vi "12-2.vi"() -> ()   [LabVIEW 2022 SP3, in "AoC22.lvlib"]
uses:
  AoC22.lvlib
  Map.ctl
panel:
  out "End gScore":i32
  out "Finished":bool
  out "No Solution":bool
  out "Elev":u8[][](graph)
  out "Cur":cluster{"Row":i32, "Col":i32}
  out "Numeric":i32
  out "Viz":i32[][](graph)
  in  "Speed":u32(slide)
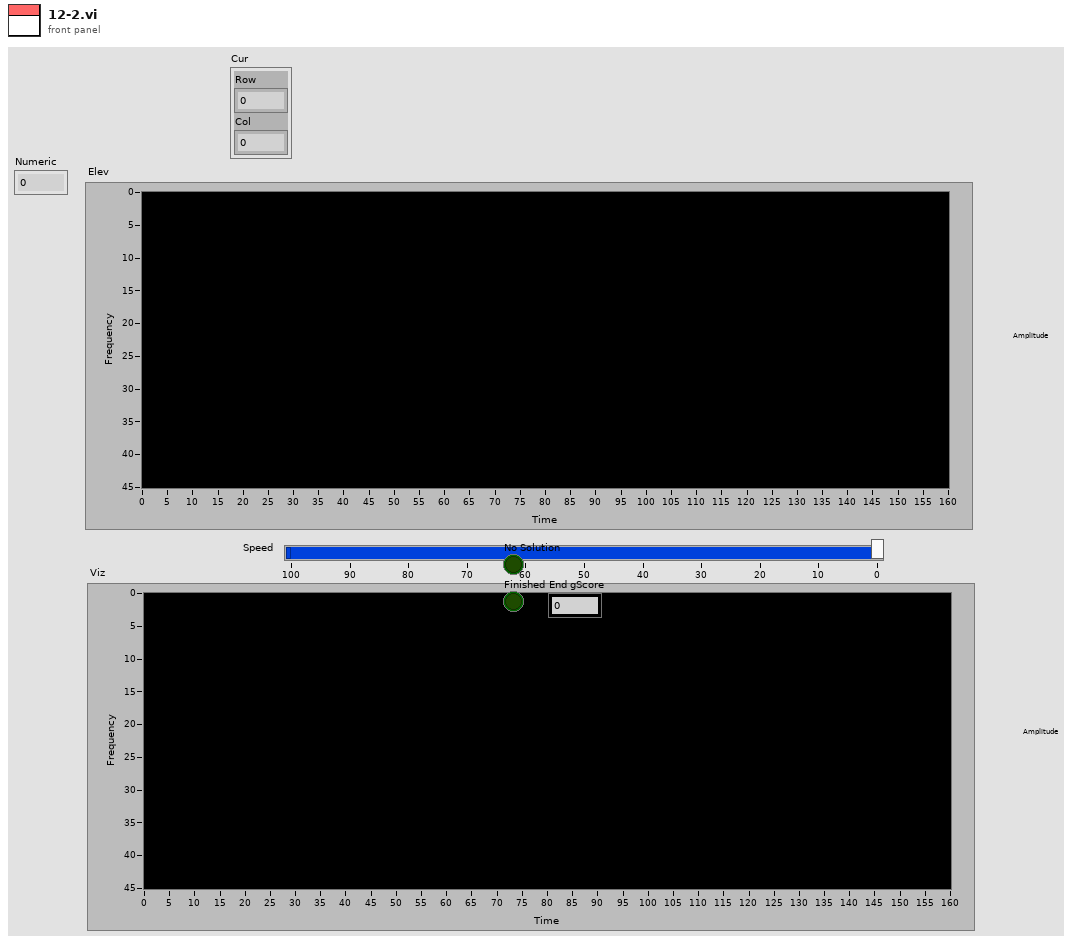
[diagram p1: front panel]
types:
  T1 = typedef "AoC22.lvlib/Map.ctl" = cluster{"Elevation":u8[][], "From":cluster{"Row":i32, "Col":i32}[][], "fScore":i32[][], "gScore":i32[][], "Start":cluster{"Row":i32, "Col":i32}, "End":cluster{"Row":i32, "Col":i32}, "openMap":map{i32, cluster{"Row":i32, "Col":i32}[]}, "openSet":set{cluster{"Row":i32, "Col":i32}}, "Vis":u8[][], "In Open":bool[][]}
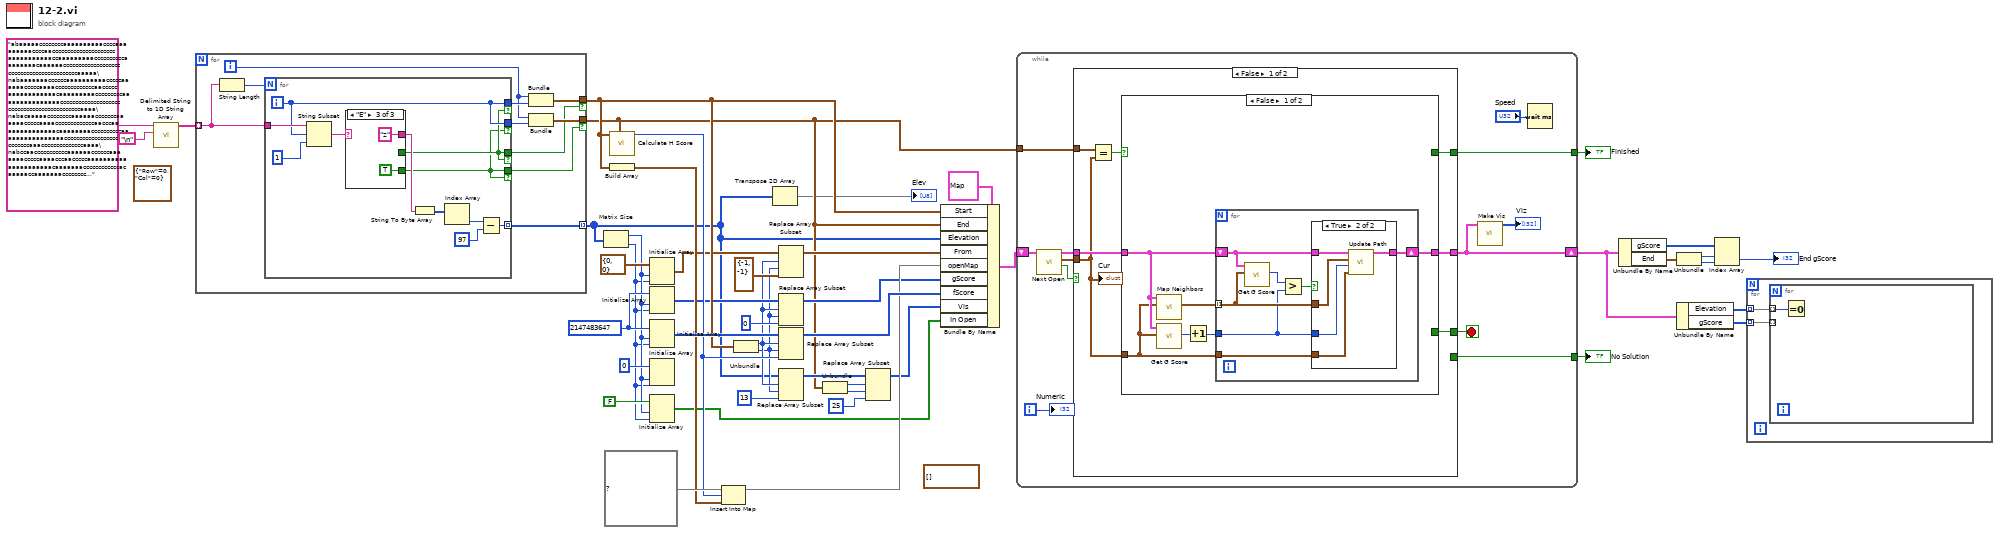
[diagram p0: block diagram]
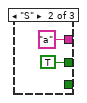
[diagram p3: hidden frame]
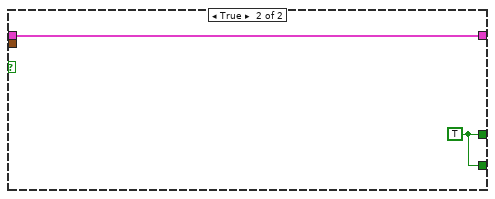
[diagram p6: hidden frame]
diagram:
  (unwired) cluster{"Row":i32, "Col":i32}[] [] ("Start")
  w37 = 2147483647 ("element")
  (unwired) cluster{"Row":i32, "Col":i32} {"Row"=0, "Col"=0}
  n1 = call <vilib>:"Delimited String to 1D String Array.vi"("delimiter"="\n", "delimited string"="abaaaaaccccccccaaaaaaaaaaccccaaaaaaaaaccccaacccccccccccccccccccccaaaaaaaaaaaccaaaaaaaaaccccccccccaaaaaaaacaaaaaaccccccccccccccccccccccccccccccccccccccccccaaaaa\nabaaaaaaaccccccaaaaaaaaaacccccaaaaaacccccaaaacccccccccccccaacccccaaaaaaaaaaaacaaaaaaaaacccccccccaaaaaaaaaaaaaaaccccccccccccccccccccccccccccccccccccccccccccaaaa\nabacaaaaaccccccccaaaaaacccccccaaaaaacccccaaaacccccccccccccaacccaaaaaaaaaaaaaacaaaaaaaaccccccccccaaaaaaaaaaaaaaaaccccccccccccccccccccccccccaaaccccccccccccccaaaa\nabccaacccccccccccaaaaaaccccccaaaaaaacccccaaaacccaacccccaaaaaaaaaaaaaaaaaaaaacaaaaaaaccccccccccccacaaaaaccaaaaaaacccccccc...") -> ("string array"=w44:string[])  [unwired: 9 in]
  n2 = for {
    tunnel: w44 -> [w55] mode=indexing
    tunnel: [w54] -> w8 mode=indexing
    tunnel: [w50] -> w34 if=w48
    tunnel: [w49] -> w13 if=w47
    i -> [w51]
    n3 = String Length(string=w55) -> (length=w56:i32)
    n4 = for {
      N: w56 -> [_]
      tunnel: w55 -> [w67]
      tunnel: [w63] -> w53 if=w62
      tunnel: [w62] -> w48 if=w62
      tunnel: [w61] -> w47 if=w61
      tunnel: [w63] -> w52 if=w61
      tunnel: [w57] -> w54 mode=indexing
      i -> [w63]
      n5 = String Subset(string=w67, offset (0)=w63, length (rest)=1 ("length (rest)")) -> (substring=w65:string)
      n6 = case shown="\"E\"" w65 {
        selector: w65 -> [w68 _ _]
        tunnel: [w68 "a" "z"] -> w64
        tunnel: [_ TRUE _] -> w62
        tunnel: [_ _ TRUE] -> w61
        frame Default {
        }
        frame "S" {
        }
        frame "E" {
        }
      }
      n7 = String To Byte Array(string=w64) -> (unsigned byte array=w60:u8[])
      n8 = Index Array(array=w60) -> (element=w59:u8)  [unwired: 1 in]
      n9 = Subtract(x=w59, y=u8 97) -> (x-y=w57:u8)
    }
    n10 = Bundle(w51, w53) -> (w50:cluster{i32, i32})  [unwired: 1 in]
    n11 = Bundle(w51, w52) -> (w49:cluster{i32, i32})  [unwired: 1 in]
  }
  n12 = Matrix Size(0:w8) -> (1:w6:i32, 2:w5:i32)
  n13 = call "Calculate H Score.vi"("End"=w13, "Position"=w34) -> ("hScore"=w33:i32)  [unwired: 9 in]
  n14 = Build Array(w34) -> (w35:cluster{i32, i32}[])
  n15 = Initialize Array(cluster{"Row":i32, "Col":i32} {"Row"=0, "Col"=0} ("Start"), w6, w5) -> (w29:cluster{"Row":i32, "Col":i32}[][])
  n16 = Initialize Array(w37, w6, w5) -> (w21:i32[][])
  n17 = Initialize Array(w37, w6, w5) -> (w40:i32[][])
  n18 = Initialize Array(u8 0 ("element"), w6, w5) -> ()  [unwired: 1 out]
  n19 = Initialize Array(FALSE, w6, w5) -> (w4:bool[][])
  n20 = Insert Into Map(map in=map{i32, cluster{"Row":i32, "Col":i32}[]} {} ("openSet"), key=w33, value=w35) -> (map out=w32:map{i32, cluster{"Row":i32, "Col":i32}[]})  [unwired: 2 out]
  n21 = Unbundle(w34) -> (w18:i32, w17:i32)
  n22 = Transpose 2D Array(2D array=w8) -> (transposed array=→"Elev":u8[][])
  n23 = Replace Array Subset(array=w29, new element=cluster{"Row":i32, "Col":i32} {"Row"=-1, "Col"=-1} ("new element/subarray"), index (row)=w18, index (col)=w17) -> (w30:cluster{"Row":i32, "Col":i32}[][])
  n24 = Replace Array Subset(array=w21, new element=0 ("new element/subarray"), index (row)=w18, index (col)=w17) -> (w22:i32[][])
  n25 = Replace Array Subset(array=w40, new element=w33, index (row)=w18, index (col)=w17) -> (w36:i32[][])
  n26 = Replace Array Subset(array=w8, new element=u8 13 ("new element/subarray"), index (row)=w18, index (col)=w17) -> (w15:u8[][])
  n27 = Unbundle(w13) -> (w12:i32, w11:i32)
  n28 = Replace Array Subset(array=w15, new element=u8 25 ("new element/subarray"), index (row)=w12, index (col)=w11) -> (w14:u8[][])
  n29 = Bundle By Name(cluster=T1 {"Elevation"=[], "From"=[], "fScore"=[], "gScore"=[], "Start"={"Row"=0, "Col"=0}, "End"={"Row"=0, "Col"=0}, "openMap"={}, "openSet"={}, "Vis"=[], "In Open"=[]} ("Map"), "Start"=w34, "End"=w13, "Elevation"=w8, "From"=w30, "openMap"=w32, "gScore"=w22, "fScore"=w36, "Vis"=w14, "In Open"=w4) -> (w39:T1)
  n30 = while {
    shift-right: [w74] -> w3
    shift-left: w39 -> [w84]
    tunnel: [w79] -> w38
    tunnel: w13 -> [w78]
    tunnel: [w77] -> w31
    i -> [w76]
    stop <- w80 stop-if-true
    n31 = call "Next Open.vi"("Map In"=w84) -> ("Empty?"=w83:bool, "Position"=w82:cluster{"Row":i32, "Col":i32}, "Map"=w81:T1)  [unwired: 8 in]
    n32 = case shown="False" w83 {
      tunnel: w82 -> [w85 _]
      tunnel: w81 -> [w89 w114]
      tunnel: [w86 w113] -> w80
      tunnel: [w87 w114] -> w74
      tunnel: [_ w113] -> w79
      tunnel: w78 -> [w91 _]
      tunnel: [w88 _] -> w77
      frame False {
        n33 = Equal?(x=w91, y=w85) -> (x = y?=w90:bool)
        n34 = case shown="False" w90 {
          selector: w90 -> [_ w111]
          tunnel: w89 -> [w96 w112]
          tunnel: [_ w111] -> w88
          tunnel: [w92 w112] -> w87
          tunnel: [_ w111] -> w86
          tunnel: w85 -> [w93 _]
          frame False {
            n35 = call "Map Neighbors.vi"("Position"=w93, "Map"=w96) -> ("Neighbors"=w97:cluster{"Row":i32, "Col":i32}[])  [unwired: 9 in]
            n36 = call "Get G Score.vi"("Position"=w93, "Map"=w96) -> ("gScore"=w95:i32)  [unwired: 9 in]
            n37 = Increment(x=w95) -> (x+1=w94:i32)
            n38 = for {
              shift-right: [w99] -> w92
              shift-left: w96 -> [w100]
              tunnel: w97 -> [w102] mode=indexing
              tunnel: w94 -> [w98]
              tunnel: w93 -> [w101]
              n39 = call "Get G Score.vi"("Position"=w102, "Map"=w100) -> ("gScore"=w104:i32)  [unwired: 9 in]
              n40 = Greater?(x=w104, y=w98) -> (0:w103:bool)
              n41 = case shown="True" w103 {
                tunnel: w102 -> [_ w109]
                tunnel: w101 -> [_ w107]
                tunnel: w100 -> [w105 w110]
                tunnel: [w105 w106] -> w99
                tunnel: w98 -> [_ w108]
                frame False {
                }
                frame True {
                  n42 = call "Update Path.vi"("From"=w107, "gScore"=w108, "Position"=w109, "Map In"=w110) -> ("Map"=w106:T1)  [unwired: 7 in]
                }
              }
            }
          }
          frame True {
          }
        }
        "Cur" <- w85
      }
      frame True {
        w113 = TRUE
      }
    }
    n43 = call "Make Vis.vi"("Map"=w74) -> ("Vis"=→"Viz":i32[][])  [unwired: 10 in]
    n44 = Wait (ms)(milliseconds to wait="Speed") -> ()  [unwired: 1 out]
    "Numeric" <- w76
  }
  "No Solution" <- w38
  "Finished" <- w31
  n45 = Unbundle By Name(w3) -> ("gScore"=w26:i32[][], "End"=w27:cluster{"Row":i32, "Col":i32})
  n46 = Unbundle By Name(w3) -> ("Elevation"=w2:u8[][], "gScore"=w1:i32[][])
  n47 = Unbundle(w27) -> ("Row"=w25:i32, "Col"=w24:i32)
  n48 = Index Array(array=w26, index (row)=w25, index (col)=w24) -> (element=→"End gScore":i32)
  n49 = for {
    tunnel: w2 -> [w116] mode=indexing
    tunnel: w1 -> [w115] mode=indexing
    n50 = for {
      tunnel: w116 -> [w117] mode=indexing
      tunnel: w115 -> [_] mode=indexing
      n51 = Equal To 0?(x=w117) -> ()  [unwired: 1 out]
    }
  }
